vi "Send Configure Arbitrary Sequence [SEQ].vi"(5 "offset (0.00 V)":dbl[unit] format="%.4f", 6 "gain (1.00)":dbl=1.0 format="%.4f", 7 "Message Priority (Normal)":T1=enum."Normal", 8 "error in (no error)":errorcluster, 9 "sequence handle (0)":i32, 10 "channel name (\"CHANNEL1\")":string="CHANNEL1", 11 "Message Enqueuer":refnum<class "Message Enqueuer.lvclass">) -> (0 "error out":errorcluster, 3 "Message Enqueuer out":refnum<class "Message Enqueuer.lvclass">)   [LabVIEW 2015, in "CS++Fgen.lvlib" / "Configure Arbitrary Sequence [SEQ] Msg.lvclass"]
doc: "Sends the <B>CS++Fgen.lvlib:Configure Arbitrary Sequence [SEQ] Msg.lvclass</B> message.\n\n<B>CS++Fgen.lvlib:CS++Fgen.lvclass:Configure Arbitrary Sequence [SEQ].vi</B> Description:\n\nThis VI configures the properties of the function generator that affect arbitrary sequence generation. These properties are the arbitrary sequence handle, gain, and offset.\n\nNotes:\n\n(1) This VI is part of the IviFgenArbSeq [SEQ] extension group."
uses:
  Configure Arbitrary Sequence [SEQ] Msg.lvclass
  <vilib>/ActorFramework/Message Enqueuer/Message Enqueuer.lvclass
  <vilib>/ActorFramework/Message Enqueuer/Message Priority.ctl
  Configure Arbitrary Sequence [SEQ] Msg.lvclass/Configure Arbitrary Sequence [SEQ] Msg.ctl
  <vilib>/ActorFramework/Message Enqueuer/Message Enqueuer.lvclass/Message Enqueuer.ctl
  <vilib>/ActorFramework/Message Priority Queue/Priority Enqueue.vi
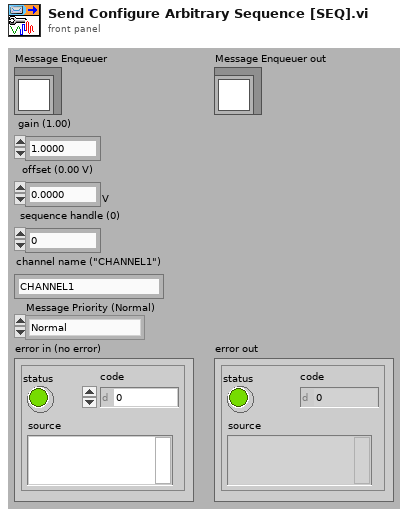
[diagram p1: front panel]
types:
  T1 = typedef "Actor Framework.lvlib/Message Enqueuer.lvclass/Message Priority.ctl" = enum16{"Low", "Normal", "High"}
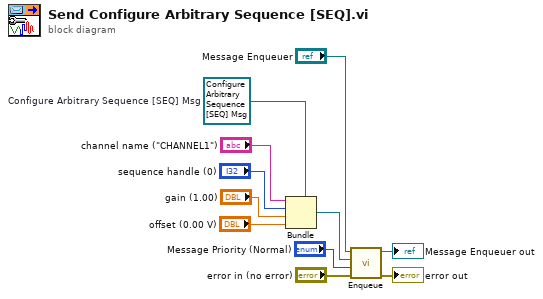
[diagram p0: block diagram]
diagram:
  w5 = refnum<class "Configure Arbitrary Sequence [SEQ] Msg.lvclass"> refnum  # Configure Arbitrary Sequence [SEQ] Msg
  n1 = Bundle(cluster=w5, "channel name (\"CHANNEL1\")", "sequence handle (0)", "gain (1.00)", "offset (0.00 V)") -> (w8:refnum<class "Configure Arbitrary Sequence [SEQ] Msg.lvclass">)
  n2 = call <vilib>:"Enqueue.vi"("error in (no error)"="error in (no error)", "Message Priority (Normal)"="Message Priority (Normal)", "Message"=w8, "Message Enqueuer in"="Message Enqueuer") -> ("error out"=→"error out":errorcluster, "Message Enqueuer out"=→"Message Enqueuer out":refnum<class "Message Enqueuer.lvclass">)  [unwired: 6 in]
